vi "GetScanPos.vi"(8 "error in (no error)":errorcluster caption="entrée d'erreur (pas d'erreur)", 11 "BaseDevice en entrée":refnum<class "BaseDevice.lvclass"> caption="DNL_LabVIEW Object in") -> (0 "error out":errorcluster caption="sortie d'erreur", 1 "Fin":dbl, 2 "nb pos":i32, 3 "BaseDevice en sortie":refnum<class "BaseDevice.lvclass"> caption="DNL_LabVIEW Object out", 4 "Increment":dbl=1.0, 6 "Debut":dbl)   [LabVIEW 2019, in "BaseDevice.lvclass"]
uses:
  BaseDevice.lvclass
  BaseDevice.lvclass/BaseDevice.ctl
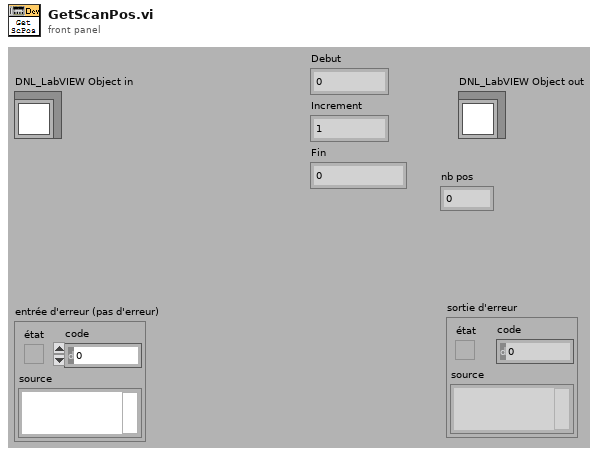
[diagram p1: front panel]
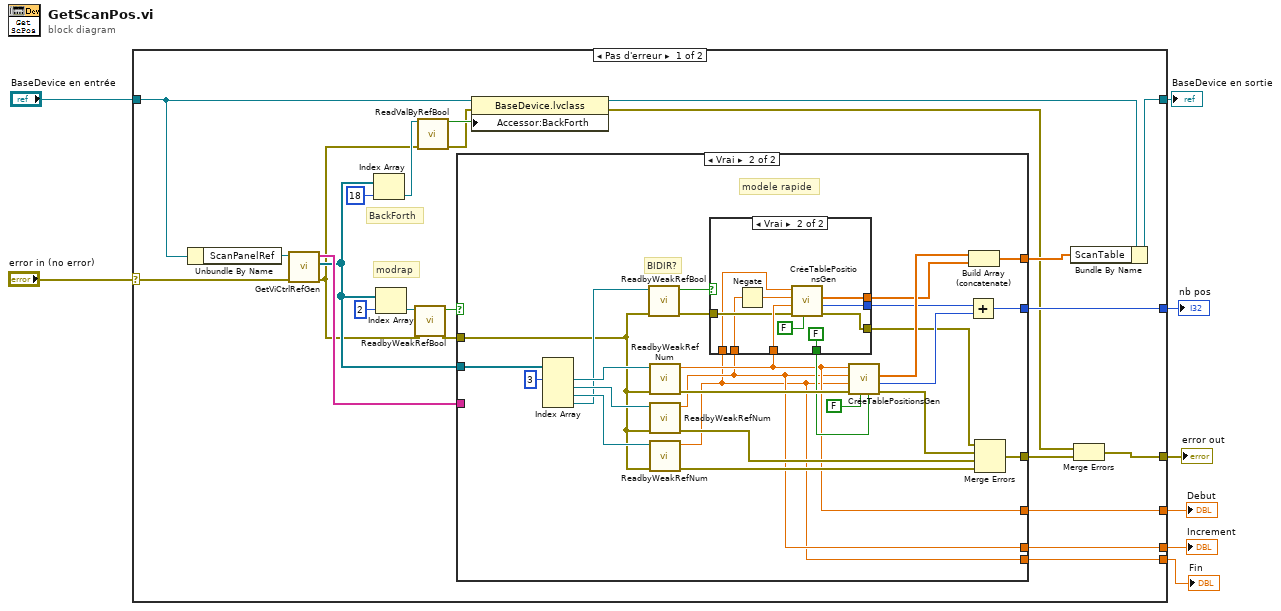
[diagram p0: block diagram]
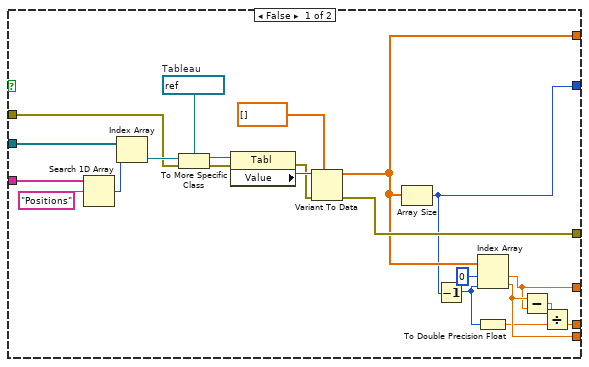
[diagram p2: hidden frame]
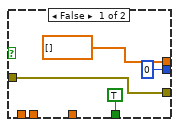
[diagram p3: hidden frame]
diagram:
  n1 = case shown="Pas d'erreur" "error in (no error)" {
    selector: "error in (no error)" -> [w27 w96]
    tunnel: [w13 w96] -> w7
    tunnel: [w24 w95] -> w5
    tunnel: "BaseDevice en entrée" -> [w32 w95]
    tunnel: [w22 _] -> w4
    tunnel: [w11 _] -> w3
    tunnel: [w10 _] -> w2
    tunnel: [w9 _] -> w1
    frame No Error {
      # "BackForth"
      # "modrap"
      n2 = Unbundle By Name(w32) -> ("ScanPanelRef"=w28:refnum<vi>)
      n3 = call <userlib>:"GetViCtrlRefGen.vi"("ErrorIn(No Error)"=w27, "VIRef"=w28) -> ("sortie d'erreur"=w15:errorcluster, "ControlsRefs"=w18:refnum<vi>[], "ControlsNames"=w21:string[])  [unwired: 7 in]
      n4 = Index Array(array=w18, index=18 ("indice")) -> (element=w16:refnum<vi>)
      n5 = Index Array(array=w18, index=2 ("indice")) -> (element=w30:refnum<vi>)
      n6 = call <userlib>:"ReadbyWeakRefBool.vi"("error in"=w15, "Control Ref"=w30) -> ("error out"=w26:errorcluster, "Valeur"=w29:bool)  [unwired: 8 in]
      n7 = call <userlib>:"ReadValByRefBool.vi"("Control Ref"=w16, "error in"=w15) -> ("Valeur"=w17:bool, "error out"=w14:errorcluster)  [unwired: 12 in]
      n8 = case shown="Vrai" w29 {
        tunnel: w18 -> [w54 w79]
        tunnel: [w41 w61] -> w23
        tunnel: w26 -> [w50 w66]
        tunnel: [w47 w70] -> w25
        tunnel: [w39 w59] -> w22
        tunnel: w21 -> [w44 _]
        tunnel: [w37 w57] -> w11
        tunnel: [w36 w56] -> w10
        tunnel: [w38 w55] -> w9
        frame False {
          w49 = refnum<vi> refnum  # Tableau
          n9 = Search 1D Array(1D array=w44, element="Positions" ("élément")) -> (index of element=w42:i32)  [unwired: 1 in]
          n10 = Index Array(array=w54, index=w42) -> (element=w53:refnum<vi>)
          n11 = To More Specific Class(target class=w49, reference=w53, error in=w50) -> (specific class reference=w52:refnum<vi>, error out=w51:errorcluster)
          n12 = property class="Tabl"(reference=w52, error in=w51) -> (error out=w46:errorcluster, "Value"=w48:variant)  [unwired: 1 out]
          n13 = Variant To Data(error in=w46, type=dbl[] [] ("ScanTable"), Variant=w48) -> (data=w41:dbl[], error out=w47:errorcluster)
          n14 = Array Size(array=w41) -> (size(s)=w39:i32)
          n15 = Decrement(x=w39) -> (x-1=w34:i32)
          n16 = Index Array(array=w41, index #1=0 ("indice"), index #2=w34) -> (element #1=w37:dbl, element #2=w38:dbl)
          n17 = To Double Precision Float(number=w34) -> (double precision float=w33:dbl)
          n18 = Subtract(x=w38, y=w37) -> (x-y=w35:dbl)
          n19 = Divide(x=w35, y=w33) -> (x/y=w36:dbl)
        }
        frame True {
          # "BIDIR?"
          # "modele rapide"
          n20 = Index Array(array=w79, index #1=3 ("indice")) -> (element #1=w78:refnum<vi>, element #2=w77:refnum<vi>, element #3=w68:refnum<vi>, element #4=w67:refnum<vi>)  [unwired: 3 in]
          n21 = call <userlib>:"ReadbyWeakRefBool.vi"("error in"=w66, "Control Ref"=w67) -> ("error out"=w65:errorcluster, "Valeur"=w64:bool)  [unwired: 8 in]
          n22 = call <userlib>:"ReadbyWeakRefNum.vi"("error in"=w66, "Control Ref"=w78) -> ("error out"=w74:errorcluster, "Valeur"=w57:dbl)  [unwired: 8 in]
          n23 = call <userlib>:"ReadbyWeakRefNum.vi"("error in"=w66, "Control Ref"=w77) -> ("error out"=w71:errorcluster, "Valeur"=w56:dbl)  [unwired: 8 in]
          n24 = call <userlib>:"ReadbyWeakRefNum.vi"("error in"=w66, "Control Ref"=w68) -> ("error out"=w72:errorcluster, "Valeur"=w55:dbl)  [unwired: 8 in]
          n25 = case shown="Vrai" w64 {
            tunnel: w57 -> [_ w94]
            tunnel: w65 -> [w83 w93]
            tunnel: w56 -> [_ w92]
            tunnel: w55 -> [_ w91]
            tunnel: [dbl[] [] ("Positions") w90] -> w60
            tunnel: [0 ("nb pos") w89] -> w58
            tunnel: [TRUE FALSE] -> w63
            tunnel: [w83 w86] -> w62
            frame False {
            }
            frame True {
              n26 = Negate(x=w92) -> (-x=w85:dbl)
              n27 = call "CréeTablePositionsGen.vi"("InvInt"=FALSE, "error in (no error)"=w93, "Fin"=w94, "Increment"=w85, "Debut"=w91) -> ("error out"=w86:errorcluster, "nb pos"=w89:i32, "Positions"=w90:dbl[])  [unwired: 4 in]
            }
          }
          n28 = call "CréeTablePositionsGen.vi"("IncFin (T)"=w63, "InvInt"=FALSE, "error in (no error)"=w74, "Fin"=w55, "Increment"=w56, "Debut"=w57) -> ("error out"=w73:errorcluster, "nb pos"=w69:i32, "Positions"=w80:dbl[])  [unwired: 3 in]
          n29 = Add(x=w58, y=w69) -> (x+y=w59:i32)
          n30 = Build Array (concatenate)(w80, w60) -> (w61:dbl[])
          n31 = Merge Errors(w62, w73, w71, w72) -> (w70:errorcluster)
        }
      }
      n32 = property class="BaseDevice.lvclass"(reference=w32, error in=w14, "Accessor:BackForth"=w17) -> (reference out=w20:refnum<class "BaseDevice.lvclass">, error out=w12:errorcluster)
      n33 = Bundle By Name(cluster=w20, "ScanTable"=w23) -> (w24:refnum<class "BaseDevice.lvclass">)
      n34 = Merge Errors(w12, w25) -> (w13:errorcluster)
    }
    frame Error {
    }
  }
  "error out" <- w7
  "BaseDevice en sortie" <- w5
  "nb pos" <- w4
  "Debut" <- w3
  "Increment" <- w2
  "Fin" <- w1
